vi "Obtain Release.vi"() -> ()   [LabVIEW 2018]
uses:
  Test Number and Bin Generator.lvclass
  Typedefs/Test Group.ctl
panel:
  in  "Test Groups":T1[](array[typedef])
  in  "Limits File Path":path
  out "error out":errorcluster
  in  "error in (no error)":errorcluster
  in  "Session  Name ()":string
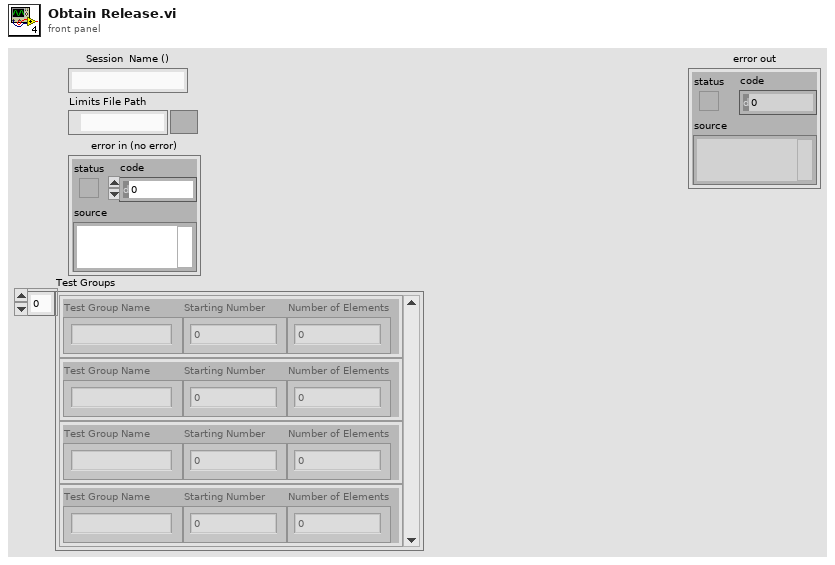
[diagram p1: front panel]
types:
  T1 = typedef "Test Number and Bin Generator.lvlib/Test Number and Bin Generator.lvclass/Test Group.ctl" = cluster{"Test Group Name":string, "Starting Number":i32, "Number of Elements":i32}
  T2 = typedef "Test Number and Bin Generator.lvlib/Test Number and Bin Generator.lvclass/Session Handle.ctl" = refnum<data-value>
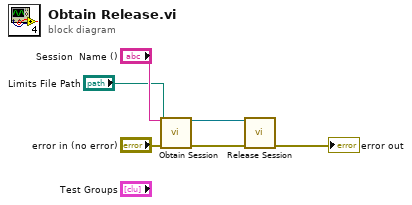
[diagram p0: block diagram]
diagram:
  n1 = call "Obtain Session.vi"("Session  Name ()"="Session  Name ()", "Limits File Path"="Limits File Path", "error in (no error)"="error in (no error)") -> ("Session Handle"=w2:T2, "error out"=w4:errorcluster)  [unwired: 11 in]
  n2 = call "Release Session.vi"("Session Handle"=w2, "error in (no error)"=w4) -> ("error out"=→"error out":errorcluster)  [unwired: 13 in]
